vi "Measure.vi"() -> ()   [LabVIEW 2013]
panel:
  out "connection ID":refnum<k5>
  out "stop":bool=TRUE
  out "_TCP disconnect":bool
  in  "TCP disconnect":bool
  out "errorOutt":errorcluster
  in  "Error":bool
  in  "SetOutput":bool
  in  "NeedToSetOutput":bool
  out "Output":string
  out "SetCurrentStr":string
  out "SetVoltageStr":string
  in  "SetVoltage":dbl format="%#.3g"
  in  "SetCurrent":dbl
  in  "NeedToSetVoltage":bool
  in  "NeedToSetCurrent":bool
  in  "Active":bool
  out "GetCurrent":string
  in  "Adress":string="172.16.21.19"
  out "GetVoltage":string
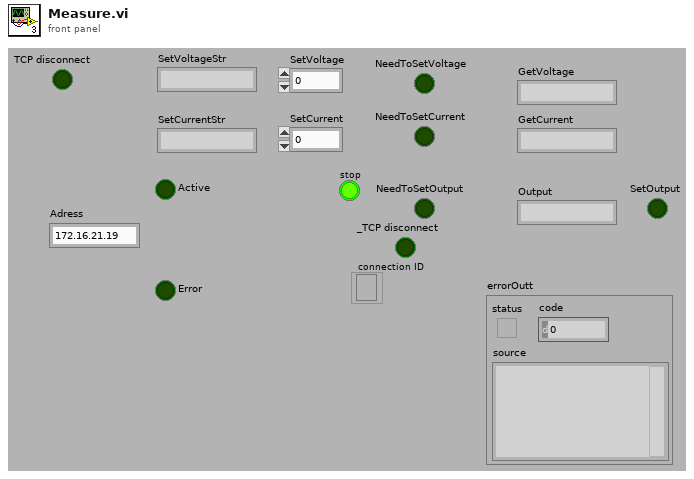
[diagram p1: front panel]
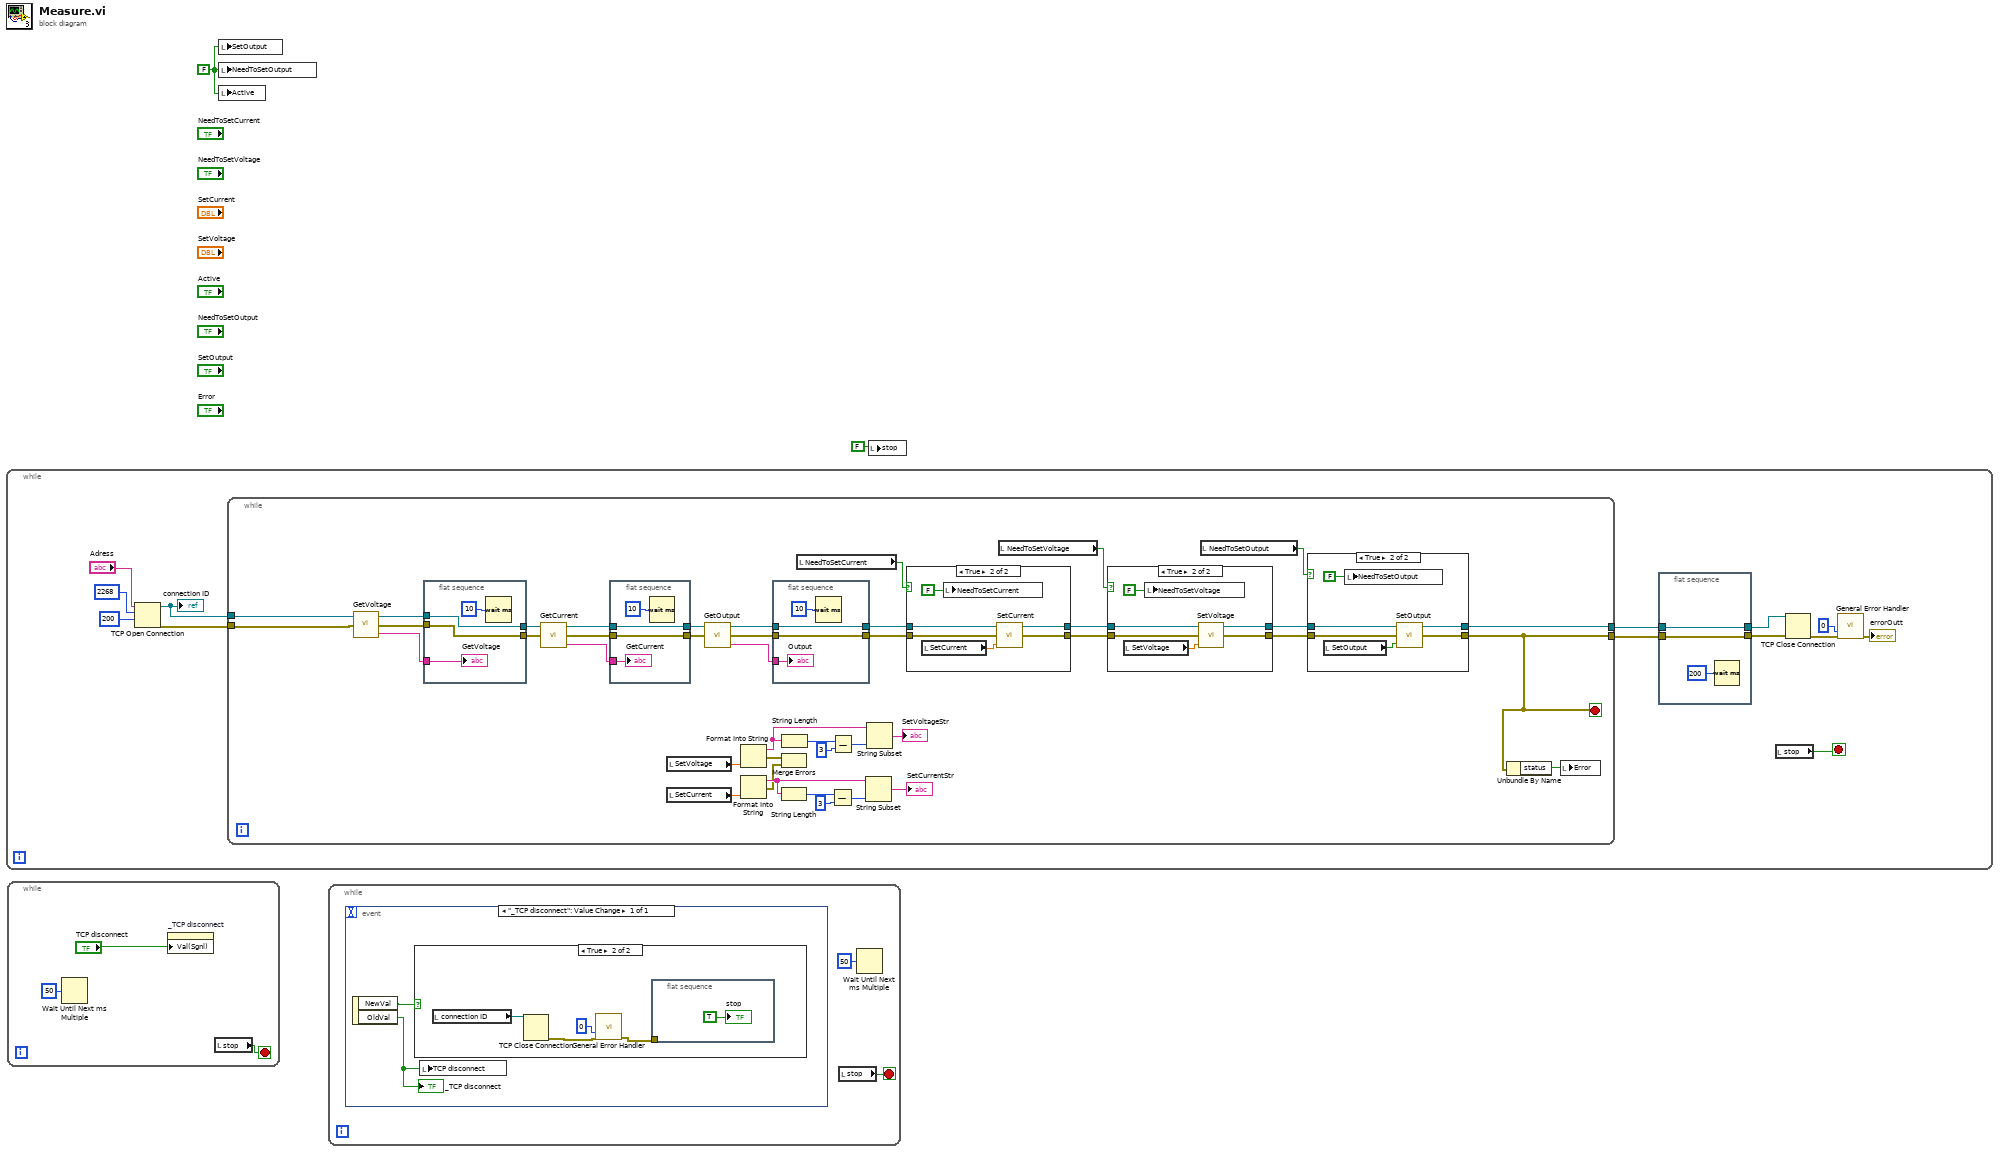
[diagram p0: block diagram]
diagram:
  w2 = FALSE ("Active")
  n1 = while {
    stop <- w3 stop-if-true
    n2 = TCP Open Connection(address="Adress", remote port or service name=u16 2268 ("Port"), timeout ms (60000)=200) -> (connection ID=w4:refnum<k5>, error out=w9:errorcluster)  [unwired: 1 in, 1 out]
    "connection ID" <- w4
    n3 = while {
      tunnel: [w19] -> w6
      tunnel: [w37] -> w7
      tunnel: w9 -> [w36]
      tunnel: w4 -> [w21]
      stop <- w19 stop-if-true
      n4 = call "GetVoltage.vi"("error in"=w36, "connection ID"=w21) -> ("Voltage"=w50:string, "error out"=w49:errorcluster, "connection ID out"=w52:refnum<k5>)  [unwired: 1 out]
      n5 = flat-sequence {
        tunnel: w52 -> [w71]
        tunnel: [w71] -> w51
        tunnel: w50 -> [w70]
        tunnel: [w69] -> w48
        tunnel: w49 -> [w69]
        frame #0 {
          n6 = Wait (ms)(milliseconds to wait=u32 10) -> ()  [unwired: 1 out]
          "GetVoltage" <- w70
        }
      }
      n7 = call "GetCurrent.vi"("error in"=w48, "connection ID"=w51) -> ("Current"=w43:string, "error out"=w47:errorcluster, "connection ID out"=w44:refnum<k5>)  [unwired: 1 out]
      n8 = flat-sequence {
        tunnel: [w67] -> w46
        tunnel: w47 -> [w67]
        tunnel: w44 -> [w66]
        tunnel: [w66] -> w45
        tunnel: w43 -> [w65]
        frame #0 {
          n9 = Wait (ms)(milliseconds to wait=u32 10) -> ()  [unwired: 1 out]
          "GetCurrent" <- w65
        }
      }
      n10 = local read "SetVoltage"() -> (w31:dbl)
      n11 = local read "SetCurrent"() -> (w30:dbl)
      n12 = call "GetOutput.vi"("error in"=w46, "connection ID"=w45) -> ("Output"=w42:string, "error out"=w41:errorcluster, "connection ID out"=w40:refnum<k5>)  [unwired: 1 out]
      n13 = Format Into String(w31) -> (resulting string=w35:string, error out=w25:errorcluster)  [unwired: 3 in]
      n14 = Format Into String(w30) -> (resulting string=w26:string, error out=w24:errorcluster)  [unwired: 3 in]
      n15 = flat-sequence {
        tunnel: [w63] -> w38
        tunnel: w41 -> [w63]
        tunnel: w40 -> [w62]
        tunnel: [w62] -> w39
        tunnel: w42 -> [w60]
        frame #0 {
          n16 = Wait (ms)(milliseconds to wait=u32 10) -> ()  [unwired: 1 out]
          "Output" <- w60
        }
      }
      n17 = Merge Errors(w25, w24) -> ()  [unwired: 1 out]
      n18 = String Length(string=w26) -> (length=w27:i32)
      n19 = String Length(string=w35) -> (length=w32:i32)
      n20 = local read "NeedToSetCurrent"() -> (w57:bool)
      n21 = Subtract(x=w27, y=3) -> (x-y=w29:i32)
      n22 = Subtract(x=w32, y=3) -> (x-y=w34:i32)
      n23 = String Subset(string=w26, length (rest)=w29) -> (substring=→"SetCurrentStr":string)  [unwired: 1 out]
      n24 = String Subset(string=w35, length (rest)=w34) -> (substring=→"SetVoltageStr":string)  [unwired: 1 out]
      n25 = case shown="True" w57 {
        tunnel: [w88 w95] -> w59
        tunnel: [w89 w92] -> w54
        tunnel: w38 -> [w89 w91]
        tunnel: w39 -> [w88 w90]
        frame False {
        }
        frame True {
          n26 = local read "SetCurrent"() -> (w93:dbl)
          n27 = local write "NeedToSetCurrent"(FALSE ("NeedToSetCurrent")) -> ()
          n28 = call "SetCurrent.vi"("Current"=w93, "error in"=w91, "connection ID"=w90) -> ("error out"=w92:errorcluster, "connection ID out"=w95:refnum<k5>)  [unwired: 1 out]
        }
      }
      n29 = local read "NeedToSetVoltage"() -> (w58:bool)
      n30 = case shown="True" w58 {
        tunnel: w59 -> [w81 w87]
        tunnel: [w81 w84] -> w56
        tunnel: w54 -> [w80 w83]
        tunnel: [w80 w82] -> w53
        frame False {
        }
        frame True {
          n31 = local read "SetVoltage"() -> (w85:dbl)
          n32 = local write "NeedToSetVoltage"(FALSE ("NeedToSetVoltage")) -> ()
          n33 = call "SetVoltage.vi"("Voltage"=w85, "error in"=w83, "connection ID"=w87) -> ("error out"=w82:errorcluster, "connection ID out"=w84:refnum<k5>)  [unwired: 1 out]
        }
      }
      n34 = local read "NeedToSetOutput"() -> (w55:bool)
      n35 = case shown="True" w55 {
        tunnel: w56 -> [w72 w77]
        tunnel: w53 -> [w73 w76]
        tunnel: [w73 w75] -> w19
        tunnel: [w72 w74] -> w37
        frame False {
        }
        frame True {
          n36 = local read "SetOutput"() -> (w78:bool)
          n37 = local write "NeedToSetOutput"(FALSE ("NeedToSetVoltage")) -> ()
          n38 = call "SetOutput.vi"("State"=w78, "error in"=w76, "connection ID"=w77) -> ("error out"=w75:errorcluster, "connection ID out"=w74:refnum<k5>)  [unwired: 1 out]
        }
      }
      n39 = Unbundle By Name(w19) -> ("status"=w20:bool)
      n40 = local write "Error"(w20) -> ()
    }
    n41 = flat-sequence {
      tunnel: [w18] -> w8
      tunnel: w7 -> [w18]
      tunnel: [w17] -> w5
      tunnel: w6 -> [w17]
      frame #0 {
        n42 = Wait (ms)(milliseconds to wait=u32 200) -> ()  [unwired: 1 out]
      }
    }
    n43 = local read "stop"() -> (w3:bool)
    n44 = TCP Close Connection(connection ID=w8, error in (no error)=w5) -> (error out=w14:errorcluster)  [unwired: 2 out]
    n45 = call <vilib>:"General Error Handler.vi"("type of dialog (OK msg:1)"=u32 0 ("millisecond multiple"), "error in (no error)"=w14) -> ("error out"=→"errorOutt":errorcluster)  [unwired: 9 in, 4 out]
  }
  n46 = while {
    stop <- w96 stop-if-true
    n47 = Wait Until Next ms Multiple(millisecond multiple=u32 50) -> ()  [unwired: 1 out]
    n48 = property on="_TCP disconnect" class="Bool (strict)"("Val(Sgnl)"="TCP disconnect") -> ()  [unwired: 2 in, 2 out]
    n49 = local read "stop"() -> (w96:bool)
  }
  n50 = local write "SetOutput"(w2) -> ()
  n51 = local write "NeedToSetOutput"(w2) -> ()
  n52 = local write "Active"(w2) -> ()
  n53 = while {
    stop <- w99 stop-if-true
    n54 = event shown="[0] \"_TCP disconnect\": Value Change" {
      selector: _ -> [_]
      dyn-events: _ -> [_]
      timeout: _ -> [_]
      event "_TCP disconnect": Value Change {
        n55 = event-data() -> ("NewVal"=w102:bool, "OldVal"=w101:bool)  [unwired: 1 in]
        "_TCP disconnect" <- w101
        n56 = case shown="True" w102 {
          frame False {
          }
          frame True {
            n57 = local read "connection ID"() -> (w103:refnum<k5>)
            n58 = TCP Close Connection(connection ID=w103) -> (error out=w104:errorcluster)  [unwired: 1 in, 2 out]
            n59 = call <vilib>:"General Error Handler.vi"("type of dialog (OK msg:1)"=u32 0 ("millisecond multiple"), "error in (no error)"=w104) -> ("error out"=w106:errorcluster)  [unwired: 9 in, 4 out]
            n60 = flat-sequence {
              tunnel: w106 -> [_]
              frame #0 {
                "stop" <- TRUE ("stop? (T)")
              }
            }
          }
        }
        n61 = local write "TCP disconnect"(w101) -> ()
      }
    }
    n62 = local read "stop"() -> (w99:bool)
    n63 = Wait Until Next ms Multiple(millisecond multiple=u32 50) -> ()  [unwired: 1 out]
  }
  n64 = local write "stop"(FALSE ("stop? (T)")) -> ()
